vi "lvCheckVI.vi"(8 "error in (no error)":errorcluster, 10 "VI Refnum":refnum<vi>, 11 "CLI":refnum<class "CLI.lvclass">) -> (0 "error out":errorcluster, 1 "Reject?":bool, 2 "dup VI Refnum":refnum<vi>, 3 "CLI out":refnum<class "CLI.lvclass">)   [LabVIEW 2014, in "lvbuildsecurity.lvlib"]
uses:
  lvbuildsecurity.lvlib
  <vilib>/Wiresmith Technology/LabVIEW CLI/CLI Class/CLI.lvclass
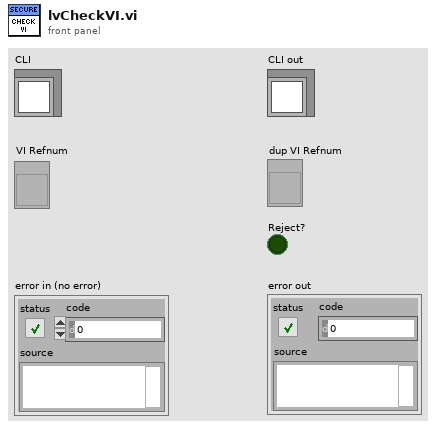
[diagram p1: front panel]
types:
  T1 = typedef "lvbuildsecurity.lvlib/ctlBlacklistClass.ctl" = cluster{"Class":string, "Items":string[]}
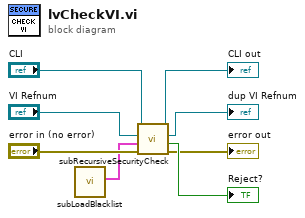
[diagram p0: block diagram]
diagram:
  n1 = call "subLoadBlacklist.vi"() -> ("Blacklist"=w6:T1[])  [unwired: 10 in, 1 out]
  n2 = call "subRecursiveSecurityCheck.vi"("error in (no error)"="error in (no error)", "Blacklist"=w6, "VI Refnum"="VI Refnum", "CLI"="CLI") -> ("error out"=→"error out":errorcluster, "Reject?"=→"Reject?":bool, "dup VI Refnum"=→"dup VI Refnum":refnum<vi>, "CLI out"=→"CLI out":refnum<class "CLI.lvclass">)  [unwired: 4 in]
